vi "Wave2D_Check Input_Domain.vi"(8 "error in (no error)":errorcluster, 11 "Domain":T1={"t"={"initial t"=0.0, "final t"=1.0, "# of t-points"=11}, "x"={"start x"=0.0, "end x"=1.0, "# of x-points"=11}, "y"={"start y"=0.0, "end y"=1.0, "# of y-points"=11}}) -> (0 "error out":errorcluster)   [LabVIEW 2017, in "NI_PDE.lvlib"]
uses:
  <vilib>/gmath/NI_PDE.lvlib
  <vilib>/gmath/pde.llb/Common/PDE_Error.ctl
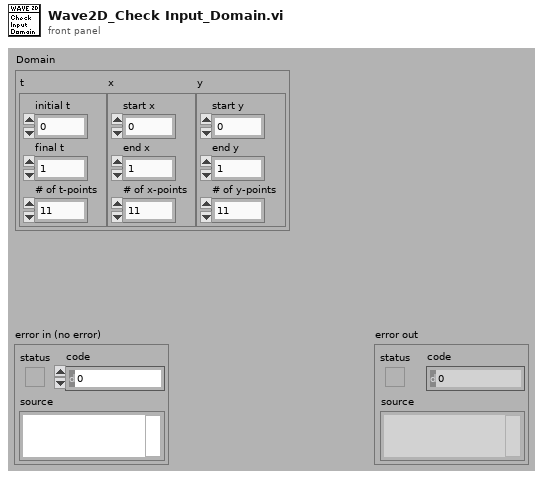
[diagram p1: front panel]
types:
  T1 = cluster{"t":cluster{"initial t":dbl, "final t":dbl, "# of t-points":i32}, "x":cluster{"start x":dbl, "end x":dbl, "# of x-points":i32}, "y":cluster{"start y":dbl, "end y":dbl, "# of y-points":i32}}
  T2 = typedef "NI_PDE.lvlib/PDE_Error.ctl" = enum16{"No Error", "k is zero", "End point <= start point", "# of time steps < 2", "# of spatial points < 3", "# of grid < 1 for FEM", "# of boundary < 3 for FEM", "Incompatible RHS size", "Incompatible BC size", "Incompatible IC size", "PDE class conflict", "RHS class conflict", "Domain class conflict", "BC class conflict", "IC class conflict"}
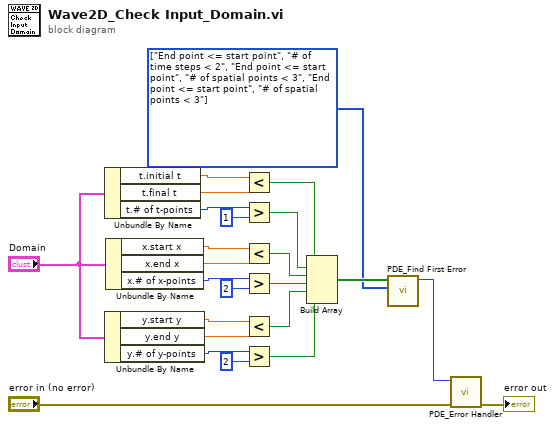
[diagram p0: block diagram]
diagram:
  w8 = T2[] [enum."End point <= start point", enum."# of time steps < 2", enum."End point <= start point", enum."# of spatial points < 3", enum."End point <= start point", enum."# of spatial points < 3"] items=["No Error", "k is zero", "End point <= start point", "# of time steps < 2", "# of spatial points < 3", "# of grid < 1 for FEM", "# of boundary < 3 for FEM", "Incompatible RHS size", "Incompatible BC size", "Incompatible IC size", "PDE class conflict", "RHS class conflict", "Domain class conflict", "BC class conflict", "IC class conflict"]
  n1 = Unbundle By Name("Domain") -> ("t.initial t"=w24:dbl, "t.final t"=w23:dbl, "t.# of t-points"=w22:i32)
  n2 = Unbundle By Name("Domain") -> ("y.start y"=w7:dbl, "y.end y"=w6:dbl, "y.# of y-points"=w5:i32)
  n3 = Unbundle By Name("Domain") -> ("x.start x"=w17:dbl, "x.end x"=w18:dbl, "x.# of x-points"=w19:i32)
  n4 = Less?(x=w24, y=w23) -> (x < y?=w16:bool)
  n5 = Greater?(x=w22, y=1) -> (0:w15:bool)
  n6 = Less?(x=w17, y=w18) -> (x < y?=w14:bool)
  n7 = Greater?(x=w19, y=2) -> (0:w13:bool)
  n8 = Less?(x=w7, y=w6) -> (x < y?=w1:bool)
  n9 = Greater?(x=w5, y=2) -> (0:w2:bool)
  n10 = Build Array(w16, w15, w14, w13, w1, w2) -> (w10:bool[])
  n11 = call <vilib>:"PDE_Find First Error.vi"("PDE Error"=w8, "Failure"=w10) -> ("first error"=w9:T2)  [unwired: 9 out]
  n12 = call <vilib>:"PDE_Error Handler.vi"("error in (no error)"="error in (no error)", "PDE error"=w9) -> ("error out"=→"error out":errorcluster)  [unwired: 9 out]
